vi "MenuHandler.vi"(5 "tree control":refnum<vi>, 7 "main queue":T1, 8 "error in":errorcluster, 9 "parameters":variant, 10 "menu string":string, 11 "CEF_serializable node in":refnum<class "CEF_serializable node.lvclass">) -> (0 "error out":errorcluster, 1 "refresh tree?":bool, 2 "Unhandled":bool, 3 "CEF_serializable node out":refnum<class "CEF_serializable node.lvclass">)   [LabVIEW 2025, in "CEF.lvlib" / "CEF_serializable node.lvclass"]
doc: "Copyright 2017 National Instruments Corporation\n\nLicensed under the Apache License, Version 2.0 (the \"License\"); you may not use this file except in compliance with the License. You may obtain a copy of the License at http://www.apache.org/licenses/LICENSE-2.0\nUnless required by applicable law or agreed to in writing, software distributed under the License is distributed on an \"AS IS\" BASIS, WITHOUT WARRANTIES OR CONDITIONS OF ANY KIND, either express or implied. See the License for the specific language governing permissions and limitations under the License."
uses:
  CEF_serializable node.lvclass
  Node/mainQref.ctl
  Node/CEF_Node.lvclass
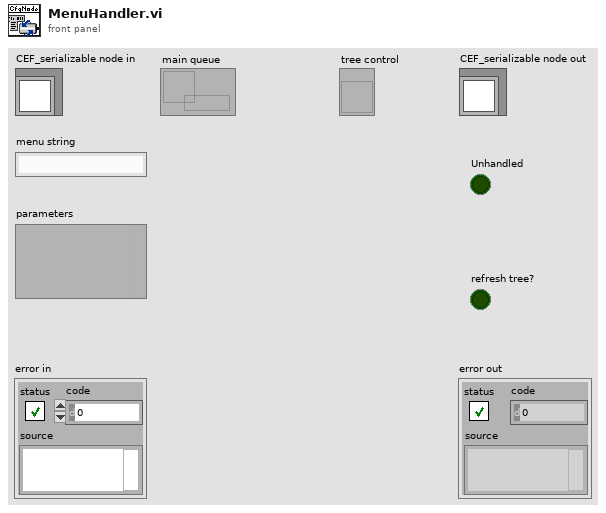
[diagram p1: front panel]
types:
  T1 = typedef "CEF.lvlib/CEF_Node.lvclass/mainQref.ctl" = refnum<queue>
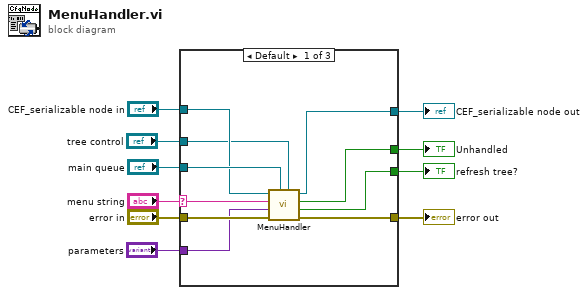
[diagram p0: block diagram]
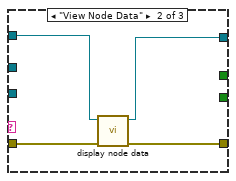
[diagram p2: hidden frame]
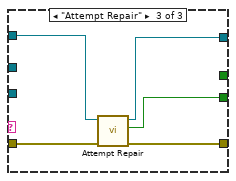
[diagram p3: hidden frame]
diagram:
  n1 = case shown="Default" "menu string" {
    selector: "menu string" -> [w12 _ _]
    tunnel: [w18 _ _] -> w6
    tunnel: "CEF_serializable node in" -> [w16 w24 w26]
    tunnel: [w15 w23 w27] -> w9
    tunnel: [w19 w22 w28] -> w5
    tunnel: "error in" -> [w20 w21 w29]
    tunnel: "main queue" -> [w17 _ _]
    tunnel: "parameters" -> [w14 _ _]
    tunnel: "tree control" -> [w13 _ _]
    tunnel: [w11 _ w25] -> w1
    frame Default {
      n2 = call-parent "MenuHandler.vi"("tree control"=w13, "main queue"=w17, "error in"=w20, "parameters"=w14, "menu string"=w12, "CEF_Node in"=w16) -> ("error out"=w19:errorcluster, "refresh tree?"=w11:bool, "Unhandled"=w18:bool, "CEF_Node out"=w15:refnum<class "CEF_serializable node.lvclass">)  [unwired: 2 in]
    }
    frame "View Node Data" {
      n3 = call-dynamic "display node data.vi"("error in"=w21, "CEF_serializable node in"=w24) -> ("error out"=w22:errorcluster, "CEF_serializable node out"=w23:refnum<class "CEF_serializable node.lvclass">)  [unwired: 8 in]
    }
    frame "Attempt Repair" {
      n4 = call "Attempt Repair.vi"("error in"=w29, "CEF_serializable node in"=w26) -> ("error out"=w28:errorcluster, "refresh tree?"=w25:bool, "CEF_serializable node out"=w27:refnum<class "CEF_serializable node.lvclass">)  [unwired: 7 in]
    }
  }
  "error out" <- w5
  "CEF_serializable node out" <- w9
  "Unhandled" <- w6
  "refresh tree?" <- w1
